vi "Result.StatusInt to String.vi"(11 "Status":T1 items=["LOG", "PASS", "FAIL", "ERROR"]) -> (3 "StatusStr":string)   [LabVIEW 2019]
uses:
  Result.Measurement and Attribute Item Status.ctl
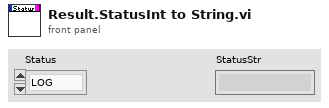
[diagram p1: front panel]
types:
  T1 = typedef "Result.Measurement and Attribute Item Status.ctl" = i32
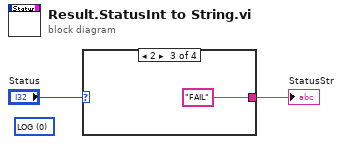
[diagram p0: block diagram]
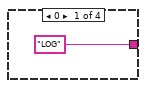
[diagram p2: hidden frame]
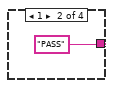
[diagram p3: hidden frame]
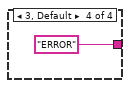
[diagram p4: hidden frame]
diagram:
  (unwired) T1 0 items=["LOG", "PASS", "FAIL", "ERROR"] ("Status")
  n1 = case shown="2" "Status" {
    tunnel: ["LOG" "PASS" "FAIL" "ERROR"] -> w1
    frame 0 {
    }
    frame 1 {
    }
    frame 2 {
    }
    frame 3, Default {
    }
  }
  "StatusStr" <- w1
